vi "ServerTCPIP_Autoguider2016.vi"() -> ()   [LabVIEW 2018]
panel:
  in  "stop":bool
  out "Status":string
  out "TCP/IP 2":bool
  out "connection ID 2":refnum<k5>
  out "serial ref":refnum<visa-resource-name>
  out "Command":string
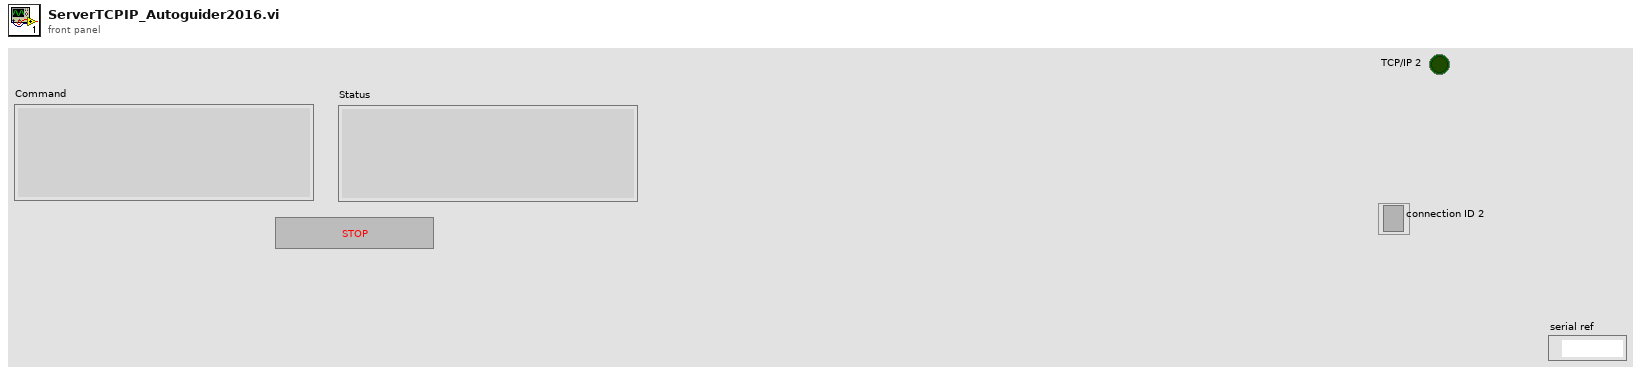
[diagram p1: front panel]
types:
  T1 = cluster{"ID":u32, "Address":string, "Service Name 1":string, "Service Name 2":string, "queue TX":refnum<queue>, "queue RX":refnum<queue>, "Port 1":u32, "Port 2":u32}
  T2 = enum16{"Standard", "Buffered", "CRLF", "Immediate"}
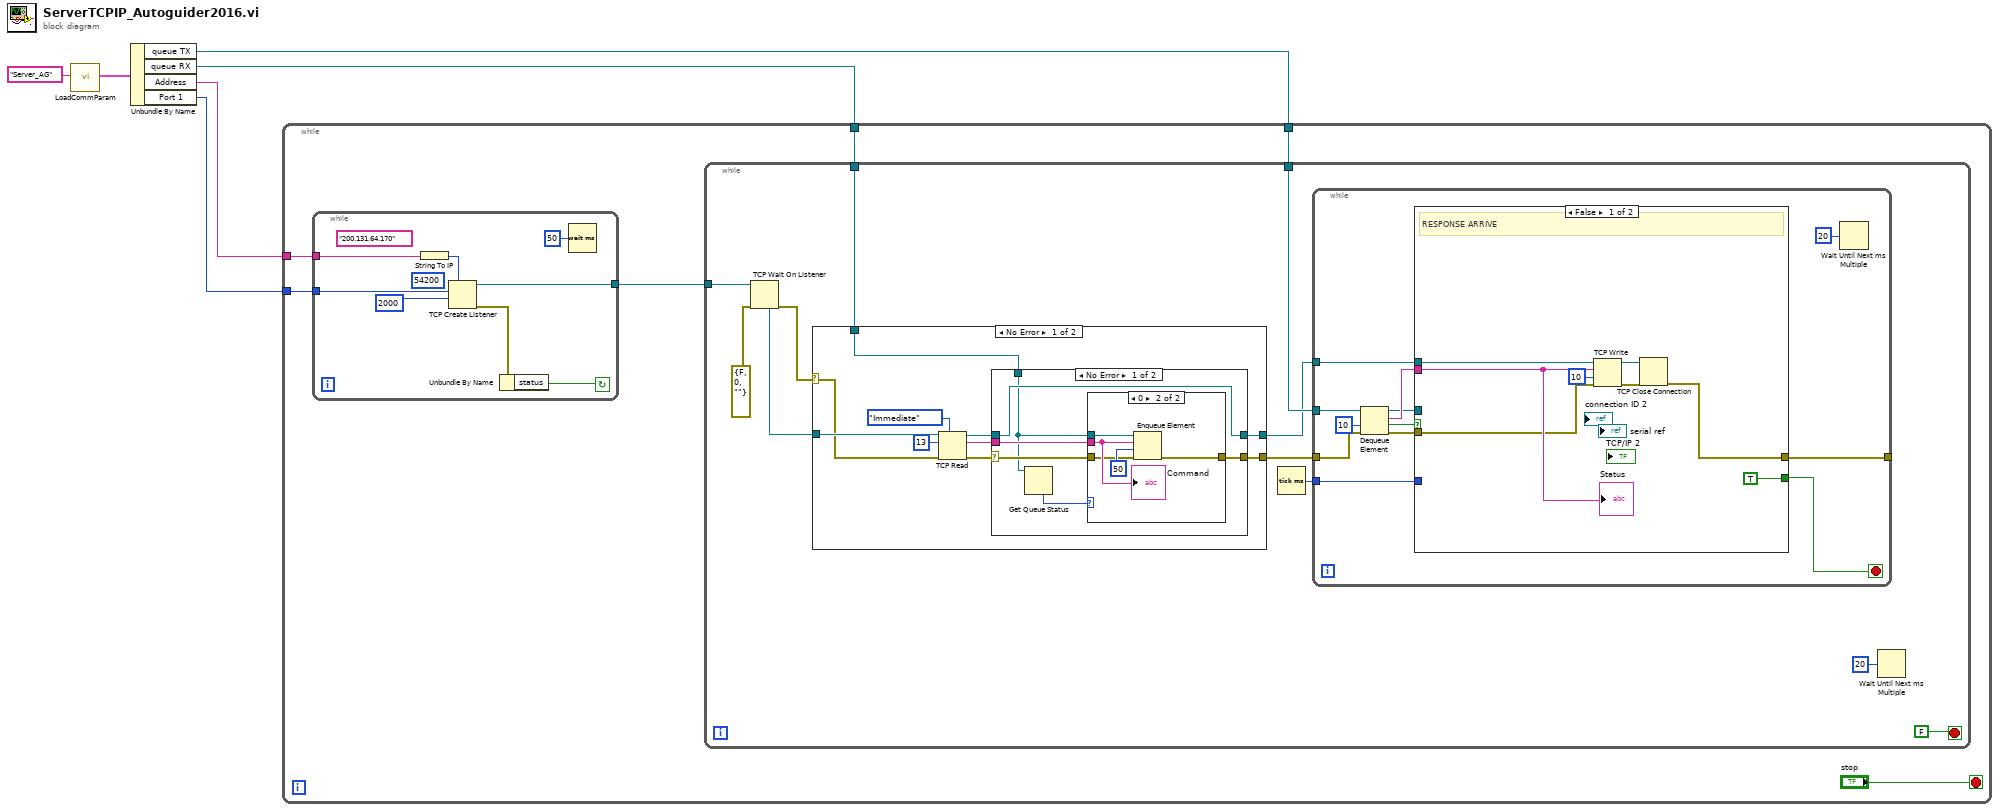
[diagram p0: block diagram]
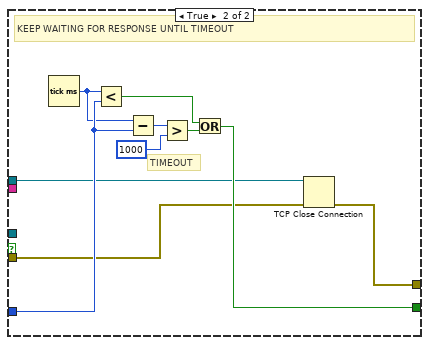
[diagram p2: hidden frame]
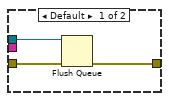
[diagram p3: hidden frame]
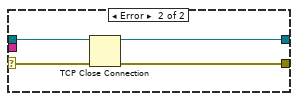
[diagram p4: hidden frame]
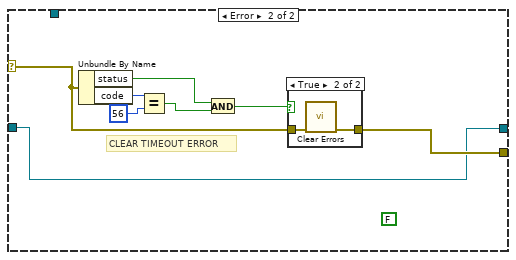
[diagram p5: hidden frame]
diagram:
  n1 = call "LoadCommParam.vi"("section name"="Server_AG") -> ("output cluster"=w5:T1)  [unwired: 10 in]
  n2 = Unbundle By Name(w5) -> ("queue TX"=w3:refnum<queue>, "queue RX"=w4:refnum<queue>, "Address"=w2:string, "Port 1"=w1:u32)
  n3 = while {
    tunnel: w4 -> [w11]
    tunnel: w3 -> [w10]
    tunnel: w2 -> [w8]
    tunnel: w1 -> [w7]
    stop <- "stop" stop-if-true
    n4 = while {
      tunnel: [w96] -> w12
      tunnel: w8 -> [w94]
      tunnel: w7 -> [w93]
      stop <- w97 continue-if-true
      (unwired) u16 54200 ("port")
      (unwired) "200.131.64.170" ("name")
      n5 = String To IP(1:w94) -> (0:w100:u32)
      n6 = TCP Create Listener(7:w100, 9:2000 ("timeout ms (25000)"), 10:w93) -> (0:w98:errorcluster, 3:w96:refnum<k5>)  [unwired: 2 in, 1 out]
      n7 = Unbundle By Name(w98) -> ("status"=w97:bool)
      n8 = Wait (ms)(milliseconds to wait=u32 50) -> ()  [unwired: 1 out]
    }
    n9 = while {
      tunnel: w12 -> [w23]
      tunnel: w11 -> [w20]
      tunnel: w10 -> [w17]
      stop <- FALSE stop-if-true
      n10 = TCP Wait On Listener(8:errorcluster {"status"=FALSE, "code"=0, "source"=""} ("error in (no error)"), 11:w23) -> (0:w21:errorcluster, 4:w22:refnum<k5>)  [unwired: 2 in, 3 out]
      n11 = case shown="No Error" w21 {
        selector: w21 -> [w56 w84]
        tunnel: w22 -> [w59 w82]
        tunnel: [w57 w83] -> w18
        tunnel: w20 -> [w58 _]
        tunnel: [w55 w82] -> w16
        frame No Error {
          n12 = TCP Read(connection ID=w59, bytes to read=13, error in (no error)=w56, 7:T2."Immediate" ("mode (standard)")) -> (connection ID out=w62:refnum<k5>, data out=w61:string, error out=w60:errorcluster)  [unwired: 1 in]
          n13 = case shown="No Error" w60 {
            selector: w60 -> [w66 w81]
            tunnel: w58 -> [w65 _]
            tunnel: [w69 w79] -> w57
            tunnel: w62 -> [w67 w80]
            tunnel: w61 -> [w68 _]
            tunnel: [w67 w78] -> w55
            frame No Error {
              n14 = Get Queue Status(queue=w65) -> (# elements in queue=w64:i32)  [unwired: 2 in, 7 out]
              n15 = case shown="0" w64 {
                tunnel: [w70 w77] -> w69
                tunnel: w68 -> [_ w76]
                tunnel: w66 -> [w71 w74]
                tunnel: w65 -> [w72 w73]
                frame Default {
                  n16 = Flush Queue(queue=w72, error in (no error)=w71) -> (error out=w70:errorcluster)  [unwired: 2 out]
                }
                frame 0 {
                  n17 = Enqueue Element(queue=w73, element=w76, timeout in ms (-1)=50, error in (no error)=w74) -> (error out=w77:errorcluster)  [unwired: 2 out]
                  "Command" <- w76
                }
              }
            }
            frame Error {
              n18 = TCP Close Connection(connection ID=w80, error in (no error)=w81) -> (connection ID out=w78:refnum<k5>, error out=w79:errorcluster)  [unwired: 1 in]
            }
          }
        }
        frame Error {
          (unwired) FALSE
          # "CLEAR TIMEOUT ERROR"
          n19 = Unbundle By Name(w84) -> ("status"=w85:bool, "code"=w89:i32)
          n20 = Equal?(x=w89, y=56 ("specific error code to clear (0: all)")) -> (x = y?=w86:bool)
          n21 = And(x=w85, y=w86) -> (x .and. y?=w87:bool)
          n22 = case shown="True" w87 {
            tunnel: w84 -> [w90 w92]
            tunnel: [w90 w91] -> w83
            frame False {
            }
            frame True {
              n23 = call <vilib>:"Clear Errors.vi"("error in (no error)"=w92) -> ("error out"=w91:errorcluster)  [unwired: 5 in, 1 out]
            }
          }
        }
      }
      n24 = Tick Count (ms)() -> (millisecond timer value=w19:u32)
      n25 = while {
        tunnel: w19 -> [w31]
        tunnel: w17 -> [w28]
        tunnel: w16 -> [w27]
        tunnel: w18 -> [w30]
        tunnel: [w29] -> _
        stop <- w32 stop-if-true
        n26 = Dequeue Element(queue=w28, timeout in ms (-1)=10, error in (no error)=w30) -> (queue out=w24:refnum<queue>, element=w35:string, timed out?=w34:bool, error out=w33:errorcluster)
        n27 = case shown="False" w34 {
          tunnel: w33 -> [w36 w46]
          tunnel: w35 -> [w41 _]
          tunnel: w31 -> [_ w53]
          tunnel: [TRUE w47] -> w32
          tunnel: [w43 w45] -> w29
          tunnel: w27 -> [w38 w44]
          tunnel: w24 -> [_ _]
          frame False {
            # "RESPONSE ARRIVE"
            n28 = TCP Write(connection ID=w38, data in=w41, error in (no error)=w36, 9:10 ("timeout ms (25000)")) -> (connection ID out=w39:refnum<k5>, error out=w40:errorcluster)  [unwired: 1 out]
            n29 = TCP Close Connection(connection ID=w39, error in (no error)=w40) -> (error out=w43:errorcluster)  [unwired: 1 in, 1 out]
            "Status" <- w41
          }
          frame True {
            # "TIMEOUT"
            # "KEEP WAITING FOR RESPONSE UNTIL TIMEOUT"
            n30 = Tick Count (ms)() -> (millisecond timer value=w52:u32)
            n31 = Less?(x=w52, y=w53) -> (x < y?=w48:bool)
            n32 = Subtract(x=w52, y=w53) -> (x-y=w51:u32)
            n33 = Greater?(x=w51, y=u32 1000 ("millisecond timer value")) -> (0:w49:bool)
            n34 = Or(x=w48, y=w49) -> (x .or. y?=w47:bool)
            n35 = TCP Close Connection(connection ID=w44, error in (no error)=w46) -> (error out=w45:errorcluster)  [unwired: 1 in, 1 out]
          }
        }
        n36 = Wait Until Next ms Multiple(millisecond multiple=u32 20) -> ()  [unwired: 1 out]
      }
      n37 = Wait Until Next ms Multiple(millisecond multiple=u32 20) -> ()  [unwired: 1 out]
    }
  }
